vi "VI-Create XControl Property Dialog.vi"() -> ()   [LabVIEW 2015]
panel:
  in  "Display State Element":u16(ring)
  out "XControl":string
  in  "Property":cluster{"Property Name":string, "Direction":u16}={"Property Name"="Property", "Direction"=0} {"Direction" items=["Read/Write", "Read only", "Write only"]}
  out "exit":bool
  in  "Create XControl":bool
  # "XControl"
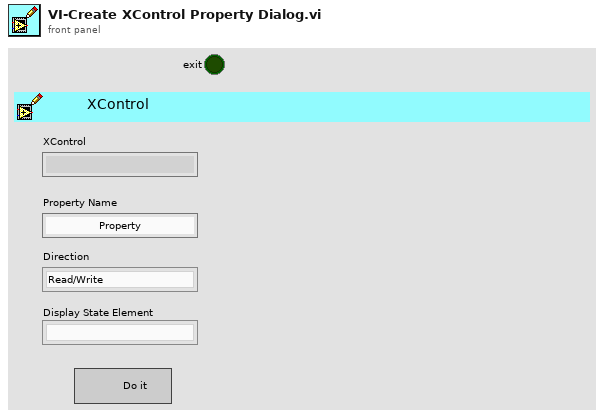
[diagram p1: front panel]
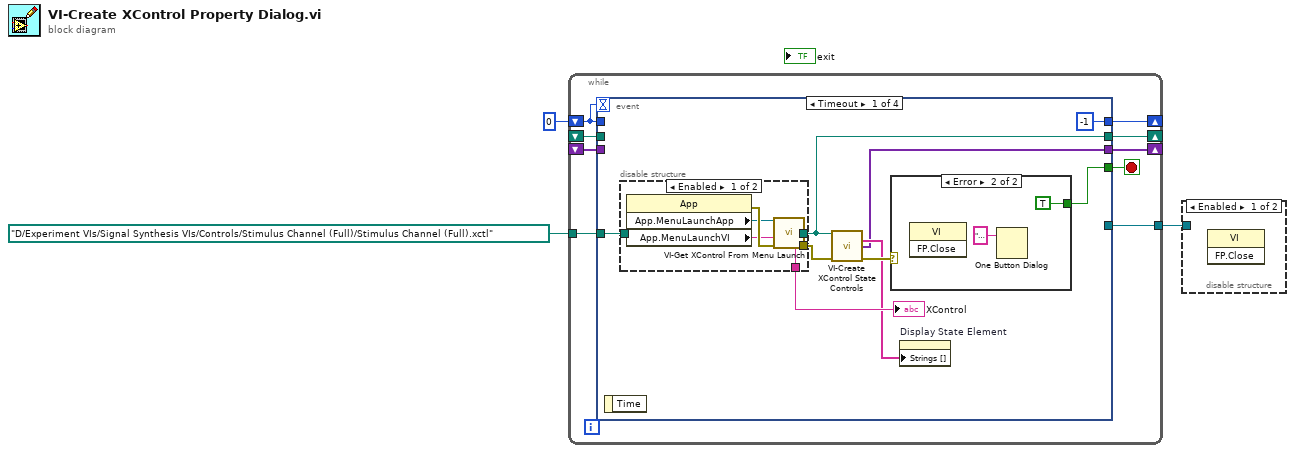
[diagram p0: block diagram]
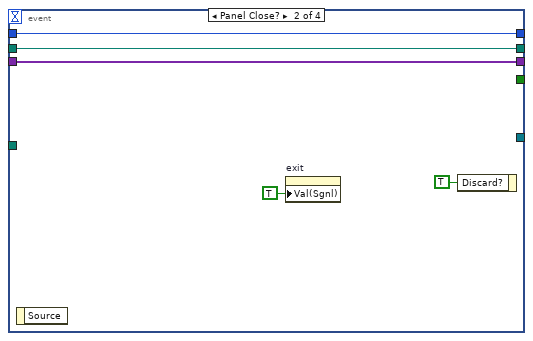
[diagram p5: hidden frame]
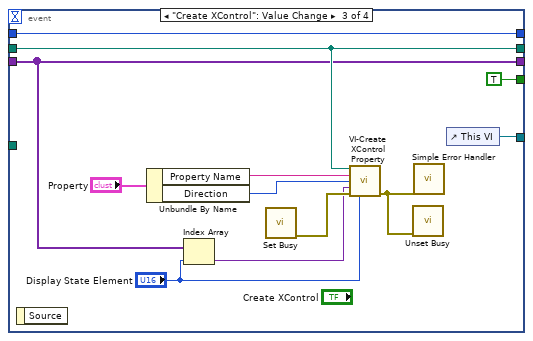
[diagram p6: hidden frame]
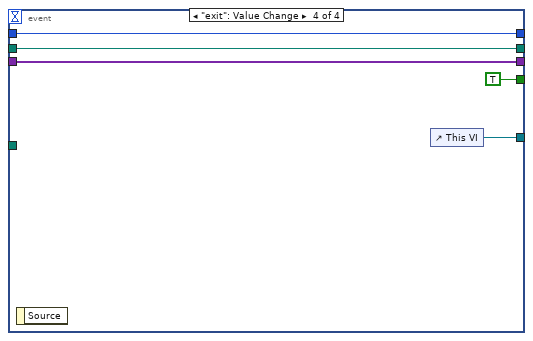
[diagram p7: hidden frame]
diagram:
  n1 = while {
    tunnel: [w12] -> w3
    shift-right: [w9] -> _
    shift-left: 0 -> [w10]
    shift-right: [w8] -> _
    shift-left: _ -> [w7]
    shift-right: [w6] -> _
    shift-left: _ -> [w5]
    tunnel: path "D:/Experiment VIs/Signal Synthesis VIs/Controls/Stimulus Channel (Full)/Stimulus Channel (Full).xctl" ("Path") -> [w4]
    stop <- w11 stop-if-true
    n2 = event shown="[0] Timeout" {
      selector: _ -> [_ _ _ _]
      dyn-events: _ -> [_ _ _ _]
      timeout: w10 -> [_ _ _ _]
      tunnel: [_ _ w46 w52] -> w12
      tunnel: [w20 _ TRUE TRUE] -> w11
      tunnel: w10 -> [_ w33 w44 w50]
      tunnel: [-1 w33 w44 w50] -> w9
      tunnel: [w17 w32 w40 w49] -> w8
      tunnel: w7 -> [_ w32 w40 w49]
      tunnel: [w14 w31 w38 w48] -> w6
      tunnel: w5 -> [_ w31 w38 w48]
      tunnel: w4 -> [w13 _ _ _]
      event Timeout {
        n3 = event-data() -> ()  [unwired: 1 in, 1 out]
        n4 = disable-structure shown="Enabled" {
          disable-tunnel: [w27 _] -> w19
          disable-tunnel: [w26 _] -> w18
          disable-tunnel: [w25 w28] -> w17
          disable-tunnel: w13 -> [_ w28]
          frame Enabled {
            n5 = property class="App"() -> (error out=w24:errorcluster, "App.MenuLaunchApp"=w22:refnum<vi>, "App.MenuLaunchVI"=w23:string)  [unwired: 2 in, 1 out]
            n6 = call "VI-Get XControl From Menu Launch.vi"("Application in"=w22, "App.MenuLaunchVI"=w23, "error in (no error)"=w24) -> ("Path"=w25:path, "Name"=w27:string, "error out"=w26:errorcluster)  [unwired: 8 in, 2 out]
          }
          frame Disabled {
          }
        }
        "XControl" <- w19
        n7 = call "VI-Create XControl State Controls.vi"("Path"=w17, "error in (no error)"=w18) -> ("Names"=w15:string[], "Data Types"=w14:variant[], "error out"=w16:errorcluster)  [unwired: 11 in]
        n8 = case shown="Error" w16 {
          tunnel: [_ TRUE] -> w20
          frame No Error {
          }
          frame Error {
            n9 = invoke class="VI" method="FP.Close"() -> ()  [unwired: 3 in, 3 out]
            n10 = One Button Dialog(message="Must create a property from the menu of one of the XControl's project items.") -> ()  [unwired: 1 in, 1 out]
          }
        }
        n11 = property on="Display State Element" class="Ring (strict)"("Strings []"=w15) -> ()  [unwired: 2 in, 2 out]
      }
      event Panel Close? {
        n12 = event-data() -> ()  [unwired: 1 in, 1 out]
        n13 = property on="exit" class="Bool (strict)"("Val(Sgnl)"=TRUE ("Value (Signaling)")) -> ()  [unwired: 2 in, 2 out]
        n14 = event-data("Discard?"=TRUE) -> ()  [unwired: 1 in, 1 out]
      }
      event "Create XControl": Value Change {
        n15 = event-data() -> ()  [unwired: 1 in, 1 out]
        n16 = Unbundle By Name("Property") -> ("Property Name"=w43:string, "Direction"=w39:u16)
        n17 = Index Array(array=w38, index="Display State Element") -> (element=w37:variant)
        n18 = call <vilib>:"Set Busy.vi"() -> ("error out"=w42:errorcluster)  [unwired: 10 in, 1 out]
        n19 = call "VI-Create XControl Property.vi"("Path"=w40, "Name"=w43, "Direction"=w39, "Data Type In"=w37, "error in (no error)"=w42, "Where"="Display State Element") -> ("error out"=w41:errorcluster)  [unwired: 9 in]
        n20 = call <vilib>:"Unset Busy.vi"("error in (no error)"=w41) -> ()  [unwired: 10 in, 1 out]
        n21 = call <vilib>:"Simple Error Handler.vi"("error in (no error)"=w41) -> ()  [unwired: 4 in, 5 out]
        n22 = control-ref of="This VI"() -> (w46:refnum<vi>)
      }
      event "exit": Value Change {
        n23 = event-data() -> ()  [unwired: 1 in, 1 out]
        n24 = control-ref of="This VI"() -> (w52:refnum<vi>)
      }
    }
  }
  n25 = disable-structure shown="Enabled" {
    disable-tunnel: w3 -> [_ _]
    frame Enabled {
      n26 = invoke class="VI" method="FP.Close"() -> ()  [unwired: 3 in, 3 out]
    }
    frame Disabled {
    }
  }
